vi "Do That Thang Core.vi"(7 "Test Executive Ref out":refnum<data-value>, 8 "error in (no error)":errorcluster, 9 "Attributes Ref":refnum<data-value>, 11 "iTest Step in":refnum<class "iTest Step.lvclass">) -> (0 "error out":errorcluster)   [LabVIEW 2019, in "Test Executive.lvlib" / "Nested Conditional in While Loop Example.lvlib" / "iTest Step.lvclass"]
uses:
  <vilib>/gpm_packages/@cs/test-executive/Source/Sandbox/Nested Conditional in While Loop Example/iTest Step/iTest Step.lvclass
  <vilib>/gpm_packages/@cs/test-executive/Source/Test Executive/ITestExecutive/ITest Executive.lvclass
  <vilib>/gpm_packages/@cs/lookup-table/Source/LookupTable/LookupTable.lvclass
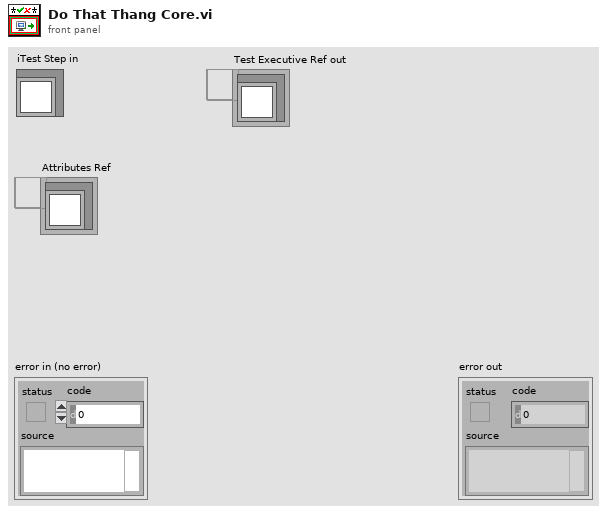
[diagram p1: front panel]
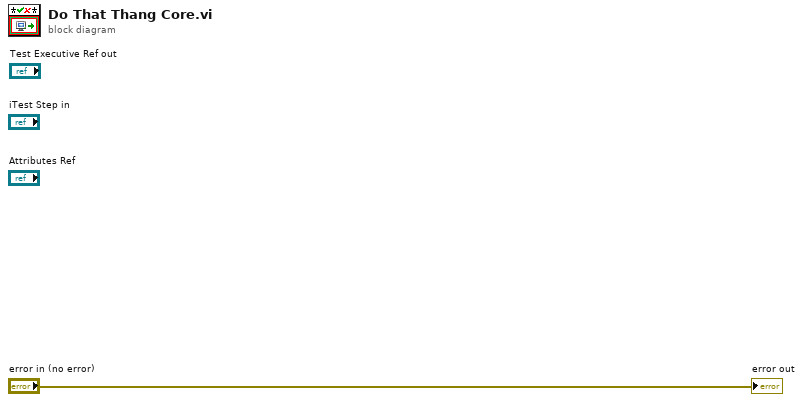
[diagram p0: block diagram]
diagram:
  "error out" <- "error in (no error)"
